vi "Wrist Teleop.vi"(11 "Wrist Toggle":bool) -> ()   [LabVIEW 2018]
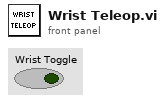
[diagram p1: front panel]
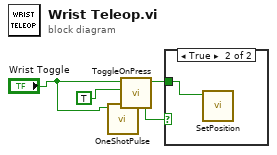
[diagram p0: block diagram]
diagram:
  n1 = call "OneShotPulse.vi"("Input"="Wrist Toggle") -> ("Output"=w2:bool)  [unwired: 10 in]
  n2 = call "ToggleOnPress.vi"("InitialOuput"=TRUE, "Input"="Wrist Toggle") -> ("Output"=w3:bool)  [unwired: 9 in]
  n3 = case shown="True" w2 {
    tunnel: w3 -> [_ w5]
    frame False {
    }
    frame True {
      n4 = call "SetPosition.vi"("Down and out?"=w5) -> ()  [unwired: 10 in, 1 out]
    }
  }
